vi "Destroy.vi"(8 "Error In":errorcluster, 11 "reference in":refnum<class "Instrument.lvclass">) -> (0 "Error Out":errorcluster, 3 "reference out":refnum<class "Instrument.lvclass">)   [LabVIEW 2023, in "HAL.lvlib" / "Instrument.lvclass"]
uses:
  Instrument.lvclass
  Instrument.lvclass/Instrument.ctl
  Configurations/CFG Base/CFG Base.lvclass
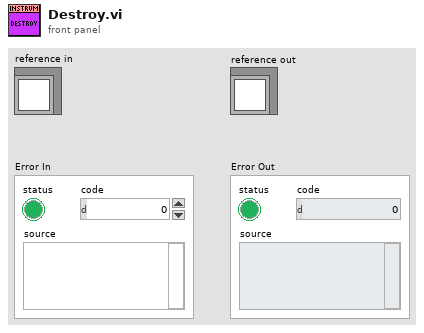
[diagram p1: front panel]
types:
  T1 = typedef "HAL.lvlib/Instrument.lvclass/ObjectAttributes.ctl" = cluster{"CFG Base":refnum<class "CFG Base.lvclass">, "Started Counter":i16}
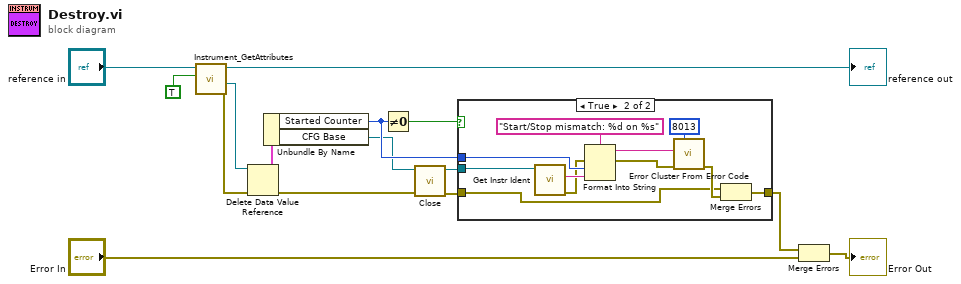
[diagram p0: block diagram]
diagram:
  n1 = call "Instrument_GetAttributes.vi"("OnlyGetDvrReference(False)"=TRUE, "reference in"="reference in") -> ("Error Out"=w12:errorcluster, "DataRef"=w11:refnum<data-value>, "reference out"=→"reference out":refnum<class "Instrument.lvclass">)  [unwired: 6 in, 1 out]
  n2 = Delete Data Value Reference(data value reference=w11, error in=w12) -> (data value=w8:T1, error out=w4:errorcluster)
  n3 = Unbundle By Name(w8) -> ("Started Counter"=w6:i16, "CFG Base"=w1:refnum<class "CFG Base.lvclass">)
  n4 = Not Equal To 0?(x=w6) -> (x != 0?=w7:bool)
  n5 = call-dynamic "Close.vi"("error in"=w4, "CFG Base in"=w1) -> ("error out"=w3:errorcluster, "CFG Base out"=w2:refnum<class "CFG Base.lvclass">)  [unwired: 8 in]
  n6 = case shown="True" w7 {
    tunnel: w3 -> [w16 w19]
    tunnel: w6 -> [_ w25]
    tunnel: [w16 w20] -> w5
    tunnel: w2 -> [_ w22]
    frame False {
    }
    frame True {
      n7 = call-dynamic "Get Instr Ident.vi"("CFG Base in"=w22) -> ("error out"=w18:errorcluster, "Instr Ident"=w21:string)  [unwired: 8 in, 1 out]
      n8 = Format Into String(format string="Start/Stop mismatch: %d on %s" ("error message (\"\")"), error in=w18, w25, w21) -> (resulting string=w24:string, error out=w17:errorcluster)  [unwired: 1 in]
      n9 = call <vilib>:"Error Cluster From Error Code.vi"("error in (no error)"=w17, "error message (\"\")"=w24, "error code (0)"=8013) -> ("error out"=w23:errorcluster)  [unwired: 6 in]
      n10 = Merge Errors(w19, w23) -> (w20:errorcluster)
    }
  }
  n11 = Merge Errors(w5, "Error In") -> (→"Error Out":errorcluster)
